vi "Cluster with a Cluster.vi"(8 "Error In":errorcluster) -> (0 "Error Out":errorcluster)   [LabVIEW 2017, in "Tests.lvlib" / "From Msgpack.lvlib"]
uses:
  From Msgpack.lvlib
  <vilib>/addons/_JKI Toolkits/Caraya/classes/Test/Test.lvclass
  src/LabPack/LabPack.lvlib
  <vilib>/addons/_JKI Toolkits/Caraya/classes/Assert/Assert.lvclass
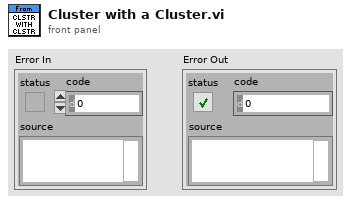
[diagram p1: front panel]
types:
  T1 = cluster{"Compact":bool, "Schema":i32, "Cluster":cluster{"Compact":bool, "Schema":i32}}
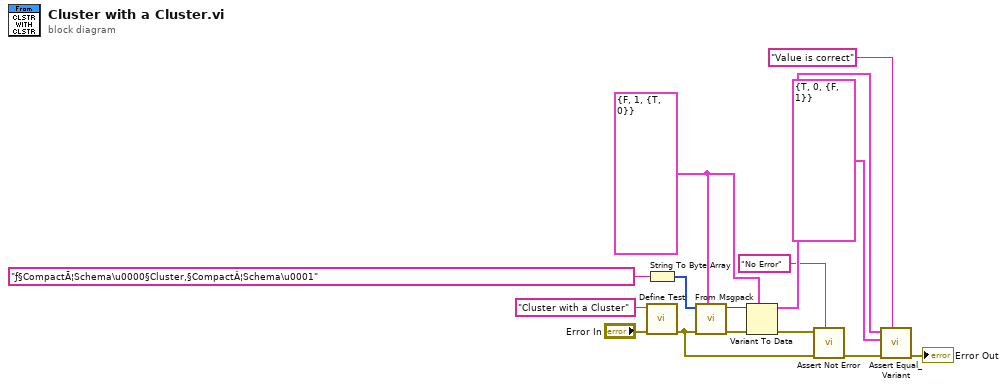
[diagram p0: block diagram]
diagram:
  w2 = T1 {"Compact"=FALSE, "Schema"=1, "Cluster"={"Compact"=TRUE, "Schema"=0}}
  n1 = String To Byte Array(string="ƒ§CompactÃ¦Schema\u0000§Cluster‚§CompactÂ¦Schema\u0001") -> (unsigned byte array=w12:u8[])
  n2 = call <vilib>:"Define Test.vi"("error in (no error)"="Error In", "Label (VI Title)"="Cluster with a Cluster") -> ("error out"=w9:errorcluster)  [unwired: 9 in]
  n3 = call "From Msgpack.vi"("Types and Defaults"=w2, "Error In"=w9, "Msgpack Data"=w12) -> ("Error Out"=w13:errorcluster, "Value"=w11:variant)  [unwired: 7 in]
  n4 = Variant To Data(error in=w13, type=w2, Variant=w11) -> (data=w6:T1, error out=w10:errorcluster)
  n5 = call <vilib>:"Assert Not Error.vi"("Label"="No Error", "error in (no error)"=w9, "Not Error?"=w10) -> ("error out"=w8:errorcluster)  [unwired: 8 in]
  n6 = call <vilib>:"Assert Equal_Variant.vi"("Label"="Value is correct", "error in (no error)"=w8, "Y"=T1 {"Compact"=TRUE, "Schema"=0, "Cluster"={"Compact"=FALSE, "Schema"=1}}, "X"=w6) -> ("error out"=→"Error Out":errorcluster)  [unwired: 7 in]
